vi "Fake Location Generator.vi"(8 "error in":errorcluster, 11 "action":T1) -> (0 "error out":errorcluster, 3 "service location":T2)   [LabVIEW 2020, in "MeasurementServerTests.lvlib" / "gRPC Utilities Tests.lvlib"]
uses:
  gRPC Utilities Tests.lvlib
  Runtime/MeasurementLink Discovery Client/RPC Messages/ni_measurementlink_discovery_v1_ServiceLocation.ctl
  Fake Location Action.ctl
  Runtime/MeasurementLink Discovery Client/MeasurementLink Discovery Client.lvlib
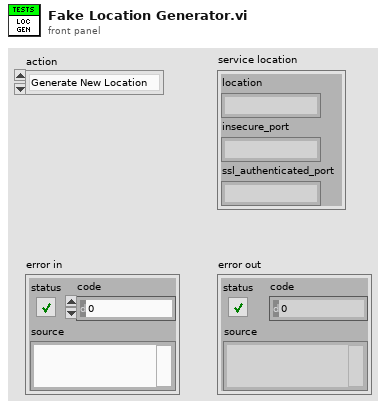
[diagram p1: front panel]
types:
  T1 = typedef "MeasurementServerTests.lvlib/gRPC Utilities Tests.lvlib/Fake Location Action.ctl" = enum16{"Generate New Location", "Reset", "Error on Next Call"}
  T2 = typedef "MeasurementLink Discovery Client.lvlib/ni_measurementlink_discovery_v1_ServiceLocation.ctl" = cluster{"location":string, "insecure_port":string, "ssl_authenticated_port":string}
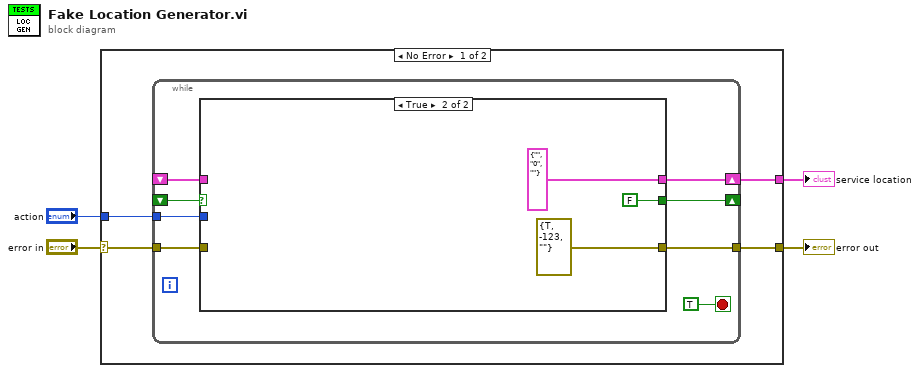
[diagram p0: block diagram]
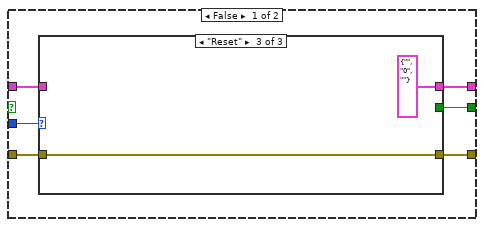
[diagram p2: hidden frame]
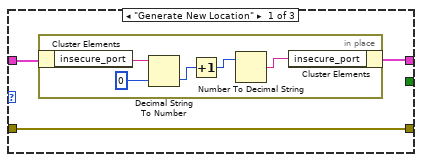
[diagram p3: hidden frame]
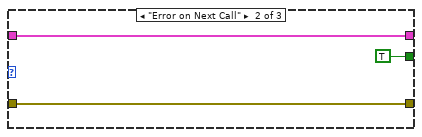
[diagram p4: hidden frame]
diagram:
  n1 = case shown="No Error" "error in" {
    selector: "error in" -> [w6 w39]
    tunnel: [w5 w39] -> w3
    tunnel: "action" -> [w8 _]
    tunnel: [w7 _] -> w2
    frame No Error {
      n2 = while {
        shift-right: [w15] -> w7
        shift-left: _ -> [w13]
        tunnel: w8 -> [w14]
        tunnel: w6 -> [w12]
        tunnel: [w11] -> w5
        shift-right: [w10] -> _
        shift-left: _ -> [w9]
        stop <- TRUE stop-if-true
        n3 = case shown="True" w9 {
          tunnel: [w22 T2 {"location"="", "insecure_port"="0", "ssl_authenticated_port"=""} ("service location")] -> w15
          tunnel: w14 -> [w21 _]
          tunnel: w13 -> [w20 _]
          tunnel: w12 -> [w19 _]
          tunnel: [w18 errorcluster {"status"=TRUE, "code"=-123, "source"=""} ("error IO")] -> w11
          tunnel: [w17 FALSE] -> w10
          frame False {
            n4 = case shown="\"Reset\"" w21 {
              tunnel: [w23 w33 T2 {"location"="", "insecure_port"="0", "ssl_authenticated_port"=""} ("service location")] -> w22
              tunnel: w20 -> [w24 w33 _]
              tunnel: w19 -> [w25 w32 w35]
              tunnel: [w25 w32 w35] -> w18
              tunnel: [_ TRUE _] -> w17
              frame "Generate New Location" {
                n5 = in-place {
                  n6 = in-place-cluster #1(w24) -> ("insecure_port"=w30:string)
                  n7 = Decimal String To Number(string=w30, default (0L)=u16 0) -> (number=w28:u16)  [unwired: 1 in, 1 out]
                  n8 = Increment(x=w28) -> (x+1=w27:u16)
                  n9 = Number To Decimal String(number=w27) -> (decimal integer string=w26:string)  [unwired: 1 in]
                  n10 = in-place-cluster #1("insecure_port"=w26) -> (w23:T2)
                }
              }
              frame "Error on Next Call" {
              }
              frame "Reset" {
              }
            }
          }
          frame True {
          }
        }
      }
    }
    frame Error {
    }
  }
  "error out" <- w3
  "service location" <- w2
